vi "UHR-Fleezers Control (host) - 12.2.vi"() -> ()   [LabVIEW 2012] (continued)
  out "Y RF Amplitude Limits (%)":T16={"Minimum"=0.0, "Maximum"=50.0, "Increment"=1.0}
  in  "Manip. X?":bool=TRUE
  in  "Manip. Y?":bool
  in  "Force Manip Abort":bool
  out "Read cal error":errorcluster
  in  "DAQ Delay (ms)":u32=1000
  in  "Start Scan":bool
  in  "Scan axis":bool=TRUE
  in  "Osc. amp. (V)":dbl=5.0
  in  "Osc. center (V)":dbl=5.0
  in  "Osc. freq. (Hz) 2":dbl=1.0
  in  "MCL Mode":u16(ring) items=["Manual Positioning", "Sinusoidal Wave", "Linear Scan"]
  in  "Begin (V)":dbl
  in  "End (V)":dbl=10.0
  in  "N Points":dbl=20.0
  in  "Delay to Interlace (s)":dbl
  in  "Delayed Interlace Start":bool
  in  "Read Lateness and Rel Phase":bool
  out "Vec Mean of T1 T2":dbl[](array[numeric])=[nan, nan]
  in  "Cal read wait (s)":u32=5
  out "Time tether formed":timestamp=timestamp(3419012832.6319866 s since 1904-01-01)
  in  "Sample Chamber Stage Serial Port":refnum<visa-resource-name>="Sample-Stage-COM1"
  in  "Chemyx Syringe Pump Serial Port":refnum<visa-resource-name>="ASRL3::INSTR"
  in  "Limit Min (MHz)":dbl=10.0 caption="Min (MHz)"
  in  "Limit Max (MHz)":dbl=16.0 caption="Max (MHz)"
  in  "Limits Enable":bool=TRUE caption="Enable"
  out "AI labels":string[](array[string])=["T1 Y", "T1 X", "T1 Sum", "T2 Y", "T2 X", "T2 Sum", "T1 FB X", "T1 FB Sum", "T2 FB X", "T2 FB Sum", "PSD Y", "PSD X", "PSD Y Sum"]
  in  "Save Trap Pos. Data":bool=TRUE
  in  "Lower Ch. Cap.":bool
  in  "Top 3 Harvard Syringe Pump Serial Port":refnum<visa-resource-name>="Top-Pump3-COM4"
  # "After"
  # "During"
  # "Trap On?"
  # "BD Flow ON?"
  # "Samp Flow ON?"
  # "Trap Trig. Fl.?"
  # "Zero It"
  # "Floor it\n(e.g., hp unwinding)"
  # "1"
  # "2"
  # "Fl. Down"
  # "Fl. Up"
  # "Bead sep"
  # "Trap Display:"
  # "APD Display:"
  # "DAQ"
  # "Data Saving"
  # "Trap Manipulation"
  # "Bead Calibration"
  # "Bottom Pump (#1)"
  # "Central Sample Channels"
  # "Top Pump (#3)"
  # "Rate param is ul/h\nVolume param is ul"
  # "Chemyx Pump 2"
  # "Units: \n1 = ml/m\n2 = ml/h\n3 = ul/m\n4 = ul/h"
  # "X"
  # "Amp switch 1st is disabled in the fpga"
  # "Y"
  # "Oscillate Set 1 freq. (debugging)"
  # "BD 1"
  # "BD 2"
  # "AOD Raster Scan"
  # "Approx. trap separations"
  # "X"
  # "Y"
  # "FPGA\nreading"
  # "DMA\ntransfer"
  # "APD Gates"
  # "APD 2"
  # "APD 1"
  # "X"
  # "2D"
  # "Y"
  # "1D"
  # "Digital Out Control"
  # "Analog Out Control (Feedback Loop)"
  # "Laser Intensity Analog Input"
  # "Analog Out Control (Feedback Loop)"
  # "Digital Out Control"
  # "Laser Intensity Analog Input"
  # "Total AI Rates (NOT rates/trap)"
  # "(Samples/trap x Trap Sets)"
  # "(Samples/channel x\n8 if averaging (8 channels)\n4 if no averaging)"
  # "Trap 1"
  # "Trap 2"
  # "Flour./Trap 3"
  # "External Video Window"
  # "MCL Position Debugging"
  # "Temporary Control Storage\n(these used to be somewhere else, still want to keep them)"
  # "Y"
  # "X"
  # "Trap Position Difference Limits"
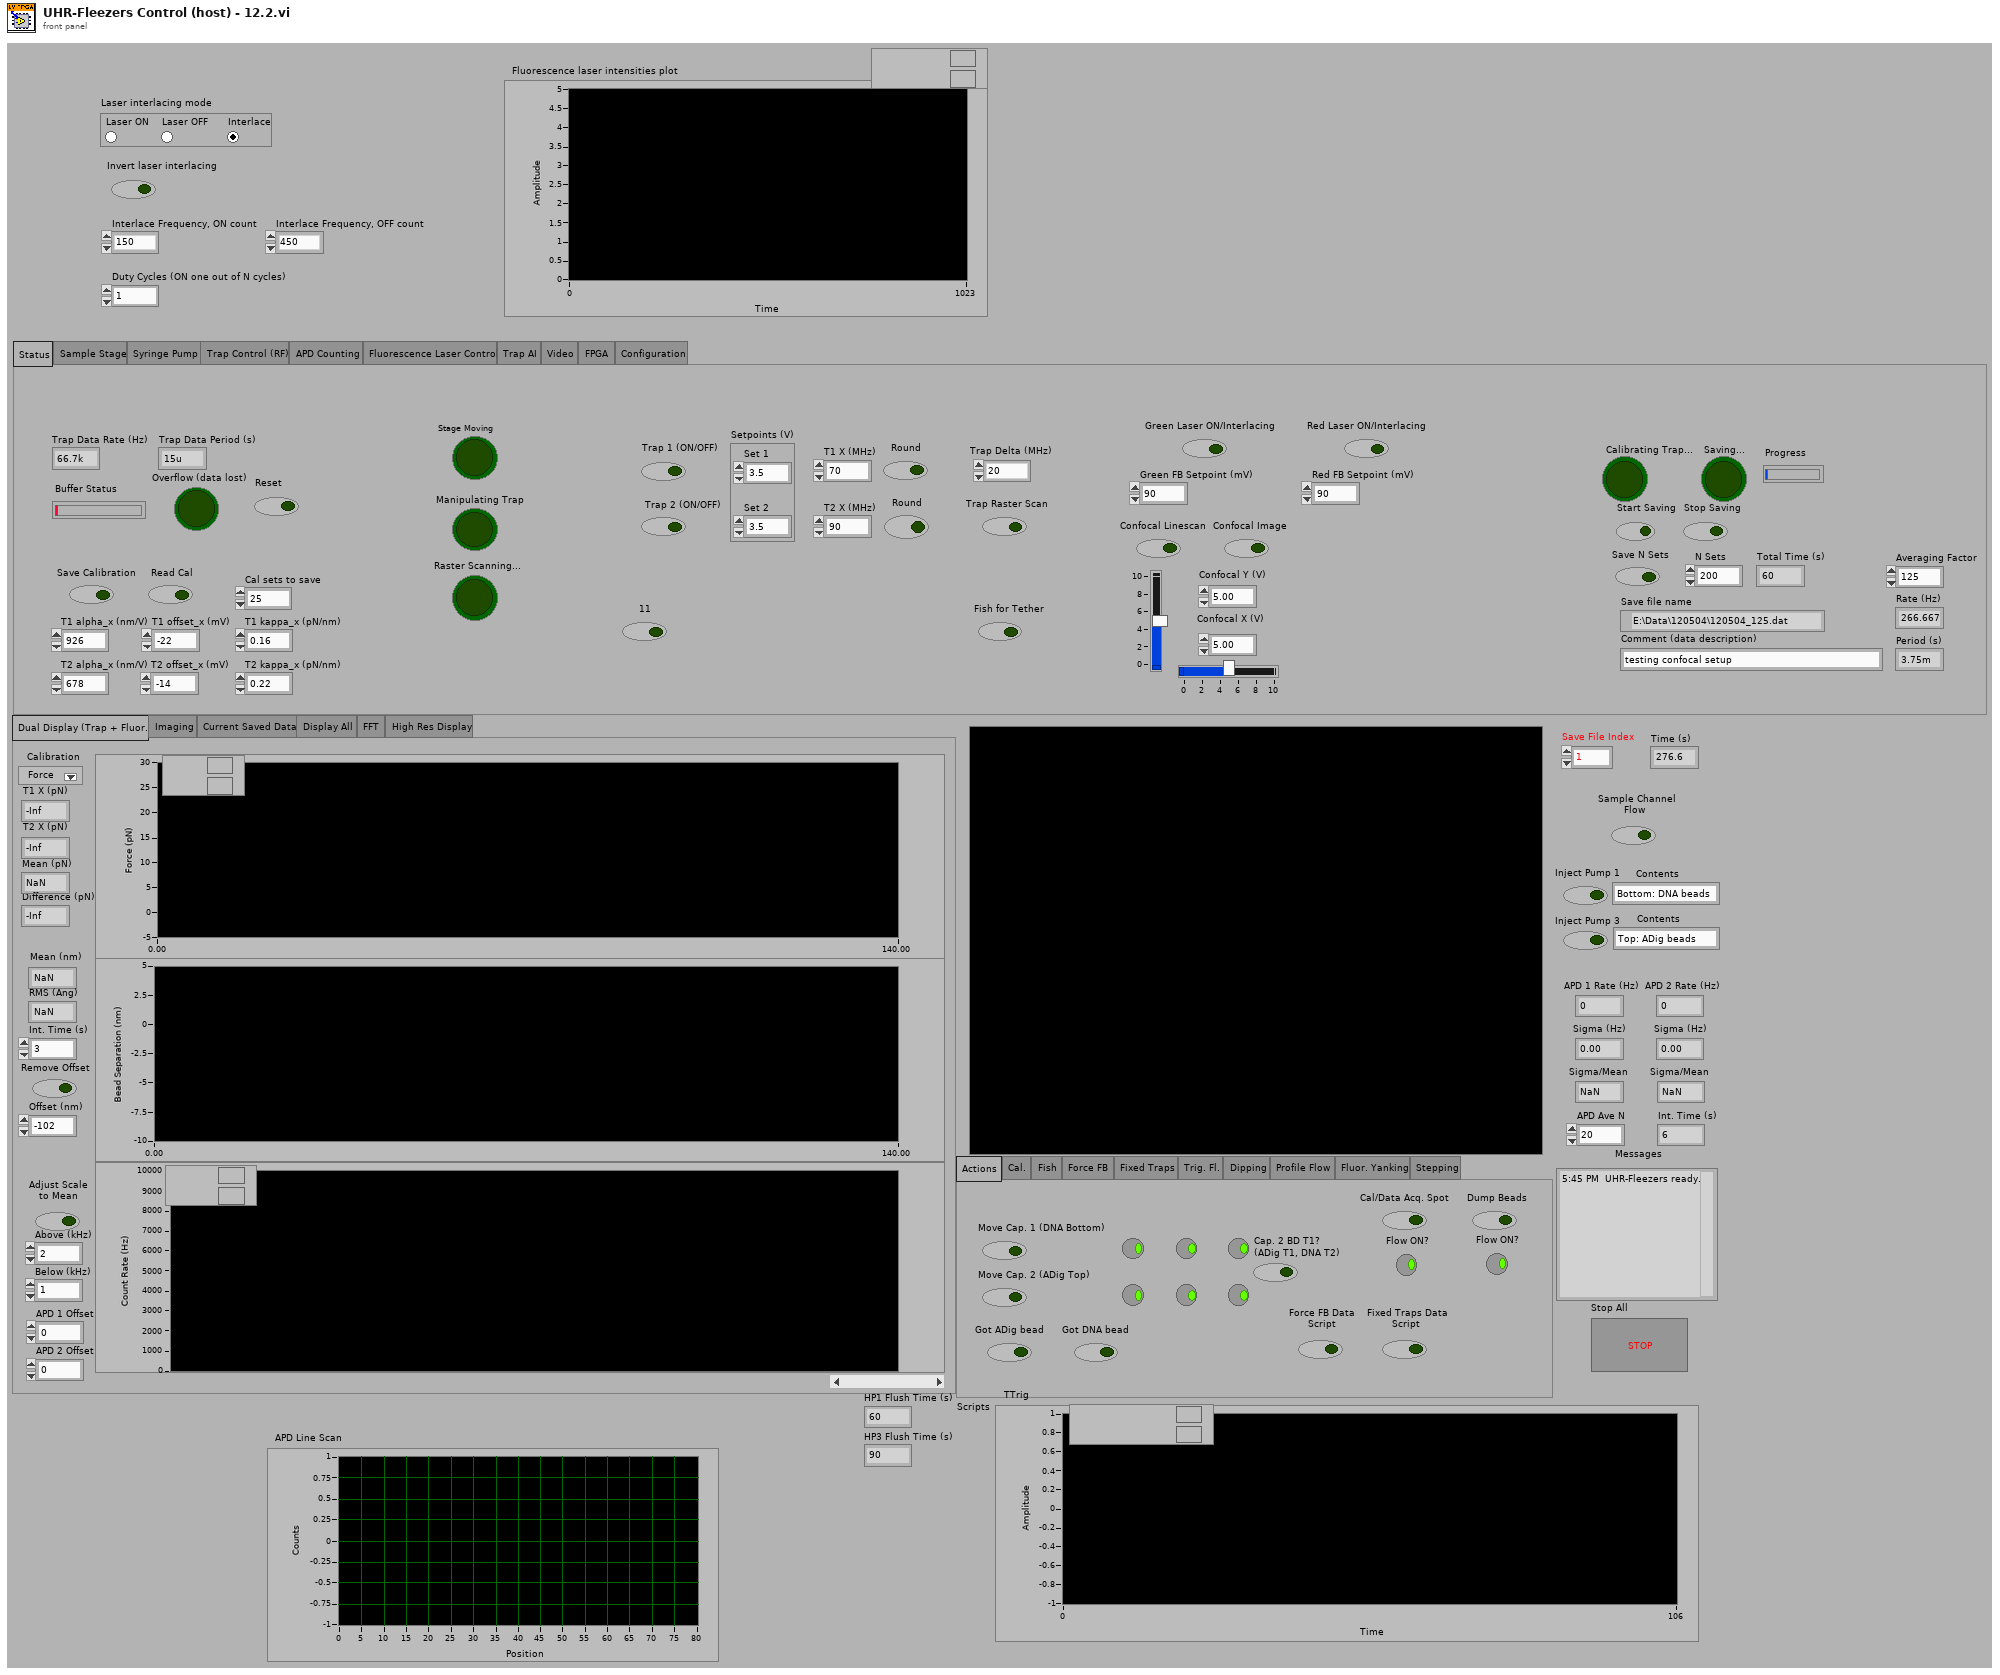
[diagram p1: front panel]
types:
  T1 = enum32{"Actions", "Cal.", "Fish", "Force FB", "Fixed Traps", "Trig. Fl.", "Dipping", "Profile Flow", "Fluor. Yanking", "Stepping"}
  T2 = typedef "IMAQ Image.ctl" = refnum<image>
  T3 = enum32{"Dual Display (Trap + Fluor.)", "Imaging", "Current Saved Data", "Display All", "FFT", "High Res Display"}
  T4 = enum32{"Status", "Sample Stage", "Syringe Pump", "Trap Control (RF)", "APD Counting", "Fluorescence Laser Control", "Trap AI", "Video", "FPGA", "Configuration"}
  T5 = cluster{"Pump 1":cluster{"Diameter (mm)":dbl, "Units":dbl, "Volume":dbl, "Rate":dbl}, "Pump 2":cluster{"Diameter (mm)":dbl, "Units":dbl, "Volume":dbl, "Rate":dbl}, "Pump 3":cluster{"Diameter (mm)":dbl, "Units":dbl, "Volume":dbl, "Rate":dbl}}
  T6 = enum32{"IR Laser Interlacing (Direct RF Board Control Method)", "AOD Raster Scan", "Feedback on Trap Intensity", "Feedback on Trap Position"}
  T7 = typedef "LVPoint32TypeDef.ctl" = cluster{"Horizontal":i32, "Vertical":i32}
  T8 = cluster{"Scan Range AOD (nm) 2":dbl, "Step Size AOD (nm) 2":dbl, "Scan Speed AOD (nm/s) 2":dbl, "Number of scans (AOD) 2":u16, "Label":string}[]
  T9 = cluster{"proportional gain (Kc)":i16, "integral gain (Kc*Ts/Ti)":i16, "derivative gain (Kc*Td/Ts)":i16}
  T10 = cluster{"Trap 1":fxp<+/-,16,1>, "Trap 2":fxp<+/-,16,1>}
  T11 = cluster{"proportional gain (Kc)":fxp<+/-,16,8>, "integral gain (Kc*Ts/Ti)":fxp<+/-,16,8>, "derivative gain (Kc*Td/Ts)":fxp<+/-,16,8>}
  T12 = cluster{"output high":fxp<+/-,16,1>, "output low":fxp<+/-,16,1>}
  T13 = cluster{"Set 1":fxp<+/-,16,1>, "Set 2":fxp<+/-,16,1>}
  T14 = enum32{"Shared Settings", "Green laser (532 nm)", "Red laser (633 nm)", "Blue laser (473 nm)"}
  T15 = cluster{"Set 1":bool, "Set 2":bool, "Set 3":bool}
  T16 = typedef "LVMinMaxIncTypeDef.ctl" = cluster{"Minimum":dbl, "Maximum":dbl, "Increment":dbl}
  T17 = typedef "Image Type" = u32
  T18 = typedef "nirio_resource_hc.ctl" = tag
  T19 = typedef "openfpgaref.8.6.ctl" = refnum<k20>
  T20 = cluster{"New Image":T2, "New Image":T2, "New Image":T2, "New Image":T2}
  T21 = typedef "XDNodeRunTimeDep.lvlib/timing_clust.ctl" = cluster{"Expected End [f-1]":u64, "Actual End [f-1]":u64, "Finished Late? [f-1]":bool, "Expected End [i-1]":u64, "Actual End [i-1]":u64, "Finished Late? [i-1]":bool, "Expected Start [i]":u64, "Actual Start [i]":u64, "Expected Start [f]":u64, "Actual Start [f]":u64, "Source Name":string, "Structure Name":string, "Period":i64, "Deadline":i64, "Offset":i64, "Start":i64, "Priority":i32, "Timeout":i32, "Mode":T22, "Wakeup Reason":T23, "Error":errorcluster, "Source Type":string, "Secondary Source Type":string, "Global End Time":u64, "Global Start Time":u64, "Frame Duration":u64, "Iteration Duration":u64, "Assigned CPU":i32, "I/O Scan Engine Mode":u32}
  T22 = typedef "XDNodeRunTimeDep.lvlib/nitl_modes.ctl" = enum32{"No Change", "Process missed periods, maintain original phase", "Discard missed periods, maintain original phase", "Process missed periods, ignore original phase", "Discard missed periods, ignore original phase"}
  T23 = typedef "XDNodeRunTimeDep.lvlib/wakeup.ctl" = enum32{"Normal", "Aborted", "Asynchronous wakeup", "Timing source error", "Timed loop error", "Timeout"}
  T24 = cluster{"Left":i32, "Top":i32, "Width":u32, "Height":u32}
  T25 = cluster{cluster{"Left":i32, "Top":i32, "Width":u32, "Height":u32}}[]
  T26 = enum32{"setting", "request", "request control", "info", "statistics", "system settings", "I/O sub system", "HRT control", "camera descriptions", "device specific data", "event sub system settings", "event sub system results", "image memory manager"}
  T27 = typedef "AviRefnum.ctl" = refnum<k1>
  T28 = typedef "imagedata.ctl" = cluster{"image type":i32, "image depth":i32, "image":u8[], "mask":u8[], "colors":u32[], "Rectangle":cluster{"left":i16, "top":i16, "right":i16, "bottom":i16}}
  T29 = enum32{"Normal Display", "Dual Display (APD)", "FFT", "High Res Display"}
  T30 = cluster{"Origin Pixel":cluster{"X":sgl, "Y":sgl}, "Angle Relative to Horizontal (deg)":sgl, "Axis Reference":u32}
  T31 = typedef "Simple Grid Descriptor" = cluster{"X Step":sgl, "Y Step":sgl, "Unit":T32}
  T32 = typedef "Image Unit" = enum32{"Undefined", "Angström", "Micrometer", "Millimeter", "Centimeter", "Meter", "Kilometer", "Microinch", "Inch", "Feet", "Nautical miles", "Standard miles", "Steps"}
  T33 = cluster{"averaging mode":u16, "weighting mode":u16, "number of averages":u32}
  T34 = cluster{"dB On (F)":bool, "unwrap phase (F)":bool, "convert to degree (F)":bool}
  T35 = enum16{"open", "replace", "create", "open or create", "replace or create", "replace or create with confirmation"}
  T36 = enum16{"big-endian, network order", "native, host order", "little-endian"}
  T37 = cluster{string, string, string, string, string, string, string, string}
  T38 = cluster{string, string, string, string, string, string, string, string, string, string, string, string}
  T39 = cluster{string, string, string, string, string, string, string, string, string, string, string, string, string}
  T40 = cluster{string, string, string, string, string, string, string, string, string, string, string, string, string, string}
  T41 = cluster{"BD 1 Frequency 1 (MHz)":dbl, "BD 1 Frequency 2 (MHz)":dbl}
  T42 = cluster{"f0":dbl, "df":dbl, "magnitude":dbl[]}[][]
  T43 = cluster{"Scan Range AOD (nm) 2":dbl, "Step Size AOD (nm) 2":dbl, "Scan Speed AOD (nm/s) 2":dbl, "Number of scans (AOD) 2":u16, "Label":string}
  T44 = cluster{"[0]":dbl, "[1]":dbl, "[2]":dbl, "[3]":dbl, "[4]":dbl, "[5]":dbl}
  T45 = cluster{"Diameter (mm)":dbl, "Units":dbl, "Volume":dbl, "Rate":dbl}
diagram:
  w58 = u16 20 items=["1.0"=10, "1.5"=15, "2.0"=20] ("stop bits (10: 1 bit)")
  w61 = u16 20 items=["1.0"=10, "1.5"=15, "2.0"=20] ("stop bits (10: 1 bit)")
  w112 = u16 20 items=["1.0"=10, "1.5"=15, "2.0"=20] ("stop bits (10: 1 bit)")
  w119 = T17 2 items=["Grayscale (U8)", "Grayscale (I16)", "Grayscale (SGL)", "Complex (CSG)", "RGB (U32)", "HSL (U32)", "RGB (U64)", "Grayscale (U16)"] ("Image Type")
  w246 = 10.0 ("y")
  w245 = 32767.0 ("y")
  w261 = 6.0  # clock mult.
  w262 = 49152000.0  # TCXO frequ.
  # "I don't think you need to do this.\nEverytime you want to adjust phase you always set this anyway.\nSince we removed the separate +/- controls.\n\nHaven't added for added fl lasers.  Should remove this code."
  # "Bottom 1 Harvard"
  # "Top 3 Harvard"
  # "Center Harvard"
  # "Bottom 1 Harvard"
  # "Top 3 Harvard"
  # "Center Harvard"
  n1 = Build Array("DIO count 1 (ticks)", "DIO count 2 (ticks)", "DIO count 3 (ticks)") -> (w166:u32[])
  n2 = local read "AO1"() -> (w240:dbl)
  n3 = local read "AO2"() -> (w239:dbl)
  n4 = local read "Scan Increment (MHz)"() -> (w257:dbl)
  n5 = local read "Continuous MCL Scanning"() -> (w227:bool)
  n6 = local read "Fast Scan Dir"() -> (w226:bool)
  n7 = local read "Number of scans (MCL)"() -> (w228:u64)
  n8 = property on="AI Count (ticks)" class="DigNum (strict)"("Val(Sgnl)"="AI Count (ticks)") -> ()  [unwired: 2 in, 2 out]
  n9 = Multiply(x=w240, y=w245) -> (x*y=w242:dbl)
  n10 = Multiply(x=w239, y=w245) -> (x*y=w244:dbl)
  n11 = Divide(x=w242, y=w246) -> (x/y=w241:dbl)
  n12 = Divide(x=w244, y=w246) -> (x/y=w243:dbl)
  n13 = To Word Integer(number=w241) -> (16bit integer=w238:i16)
  n14 = To Word Integer(number=w243) -> (16bit integer=w237:i16)
  n15 = Not(x=w226) -> (.not. x?=w221:bool)
  n16 = local read "Cycles/step (MCL)"() -> (w229:u64)
  n17 = Multiply(x=w257, y=1000.0) -> (x*y=w264:dbl)
  n18 = local read "Scan steps (MCL)"() -> (w230:u64)
  n19 = local write "Trap Pos FIFO Timeout"(u16 0 ("Trap Pos FIFO Timeout")) -> ()
  n20 = local read "Desired Scan Incr (V)"() -> (w232:dbl)
  n21 = Scale By Power Of 2(n=48, x=w264) -> (x*2^n=w265:dbl)
  n22 = Unbundle By Name(cluster{"output high":i16, "output low":i16} {"output high"=3000, "output low"=0} ("FB output range 1")) -> ("output high"=w38:i16, "output low"=w37:i16)
  n23 = Multiply(x=w262, y=w261) -> (x*y=w260:dbl)
  n24 = Divide(x=w265, y=w260) -> (x/y=w259:dbl)
  n25 = local read "Setpoints (V)"() -> (w276:cluster{"Set 1":dbl, "Set 2":dbl})
  n26 = To Quad Integer(1:w259) -> (0:w256:i64)
  n27 = Divide(x=40000000.0, y="AI Count (ticks)") -> (x/y=w217:dbl)
  n28 = Multiply(x=w232, y=32767.0) -> (x*y=w234:dbl)
  n29 = local read "Trap Intensity PID Gains"() -> (w271:T9)
  n30 = local read "Number Interlace Sets"() -> (w159:u8)
  n31 = Split 1D Array(array=w166, index=w159) -> (first subarray=w168:u32[])  [unwired: 1 out]
  n32 = Add Array Elements(numeric array=w168) -> (sum=w167:u32)
  n33 = local read "# Samples/channel"() -> (w249:u32)
  n34 = local read "Number of F/B Scans (AOD)"() -> (w250:u16)
  n35 = local read "Not-Interlacing Set"() -> (w158:enum32{"Set 1", "Set 2", "Set 3"})
  n36 = To Unsigned Byte Integer(number=w158) -> (unsigned 8bit integer=w164:u8)
  n37 = Index Array(array=w166, index=w164) -> (element=w165:u32)
  n38 = local read "Feedback On/Off"() -> (w279:cluster{"Set 1":bool, "Set 2":bool})
  n39 = local read "Scan steps (AOD)"() -> (w255:u64)
  n40 = local read "All FB On/Off"() -> (w280:bool)
  n41 = local read "Cycles/step (AOD)"() -> (w254:u64)
  n42 = local write "AI rate (Hz)"(w217) -> ()
  n43 = Divide(x=w234, y=10.0) -> (x/y=w233:dbl)
  n44 = Multiply(x=w255, y=w254) -> (x*y=w253:u64)
  n45 = Unbundle By Name(w271) -> ("proportional gain (Kc)"=w42:i16, "integral gain (Kc*Ts/Ti)"=w41:i16, "derivative gain (Kc*Td/Ts)"=w40:i16)
  n46 = Multiply(x=3276.7, y=w276) -> (x*y=w275:cluster{"Set 1":dbl, "Set 2":dbl})
  n47 = xnode "Open FPGA VI Reference"("resource name"=T18 "750kHzDAQ") -> ("FPGA VI Reference Out"=w270:T19, "error out"=w269:errorcluster)  [unwired: 1 in]
  n48 = To Word Integer(number=w233) -> (16bit integer=w231:i16)
  n49 = Multiply(x=w253, y=u64 2) -> (x*y=w251:u64)
  n50 = Divide(x=w217, y="FPGA Ave.") -> (x/y=w218:dbl)
  n51 = To Word Integer(number=w275) -> (16bit integer=w274:cluster{"Set 1":i16, "Set 2":i16})
  n52 = Multiply(x=w251, y=w250) -> (x*y=w248:u64)
  n53 = local read "Sets to FIFO (Traps)"() -> (w46:T15)
  n54 = local write "Ave. Rate (Hz)"(w218) -> ()
  n55 = Divide(x=w248, y=w249) -> (x/y=w247:dbl)
  n56 = Unbundle By Name(w274) -> ("Set 1"=w273:i16, "Set 2"=w272:i16)
  n57 = local read "2D or 1D Scan"() -> (w178:bool)
  n58 = local write "Data points/scans"(w248) -> ()
  n59 = local read "Scan BD"() -> (w266:bool)
  n60 = And(x=w279, y=w280) -> (x .and. y?=w278:cluster{"Set 1":bool, "Set 2":bool})
  n61 = local write "Data points/scan (f/b)"(w251) -> ()
  n62 = Reciprocal(x=w218) -> (1/x=w219:dbl)
  n63 = local read "N Acq Sets (Traps + Fl.)"() -> (w210:i16)
  n64 = local write "N sets should be saved"(w247) -> ()
  n65 = xnode "Invoke Method"("FPGA VI Reference In"=w270, "error in"=w269) -> ("FPGA VI Reference Out"=w177:T19, "error out"=w186:errorcluster)
  n66 = Unbundle By Name(w278) -> ("Set 1"=w282:bool, "Set 2"=w281:bool)
  n67 = local read "Interlace"() -> (w160:bool)
  n68 = Select(t=w167, s=w160, f=w165) -> (s? t:f=w157:u32)
  n69 = local write "Update Count (MCL)"(w157) -> ()
  n70 = local write "Total Counts (ticks)"(w157) -> ()
  n71 = local write "Ave. Period (s)"(w219) -> ()
  n72 = Unbundle By Name(w46) -> ("Set 1"=w45:bool, "Set 2"=w44:bool, "Set 3"=w43:bool)
  n73 = property on="2D or 1D Scan" class="Bool (strict)"("Val(Sgnl)"=w178) -> ()  [unwired: 2 in, 2 out]
  n74 = local read "Interlace Frequency, OFF count"() -> (w4:u32)
  n75 = local read "Interlace Frequency, ON count"() -> (w5:u32)
  n76 = local read "APD Gate OFF Count"() -> (w84:u32)
  n77 = local read "APD Gate ON Count"() -> (w80:u32)
  n78 = xnode "Read/Write Control"("FPGA VI Reference In"=w176, "error in"=w186, "ai count"="AI Count (ticks)", "Interlace ON/OFF"=w160, "Number Interlace Cycles"=w159, "Set 1"=w45, "Set 2"=w44, "Set 3"=w43, "FB On/Off Set 1"=w282, "FB On/Off Set 2"=w281, "Interlace Off Parameters"=w158, "FB Setpoint Set 1"=w273, "FB Setpoint Set 2"=w272, "P1"=w42, "I1"=w41, "D1"=w40, "FB1 output high"=w38, "FB1 output low"=w37, "Cycles per step"=w254, "Scan BD"=w266, "Number of scans"=w250, "Scan steps"=w255, "Scan freq.  increment"=w256, "AO1"=w238, "AO2"=w237, "Scan freq.  increment (MCL)"=w231, "Scan steps (MCL)"=w230, "Cycles per step (MCL)"=w229, "Number of scans (MCL)"=w228, "MCL count"=w157, "Cont. Scan (MCL)"=w227, "MCL Scan Axis"=w221, "1D or 2D Scan?"=w178, "N of AI1 Int Acq Sets"=w210, "Amp switch delay"="Amp switch delay", "Swap F1 and F2"="Swap F1 and F2", "APD to FIFO"=FALSE, "DIO count 1 (ticks)"="DIO count 1 (ticks)", "DIO count 2 (ticks)"="DIO count 2 (ticks)", "DIO count 3 (ticks)"="DIO count 3 (ticks)") -> ("FPGA VI Reference Out"=w90:T19, "error out"=w88:errorcluster)  [unwired: 1 in]
  n79 = local read "Duty Cycles (ON one out of N cycles)"() -> (w86:u32)
  n80 = local read "APD Integration Time (s)"() -> (w72:dbl)
  n81 = local read "DMA Update Period (s)"() -> (w71:dbl)
  n82 = Add(x=w80, y=w84) -> (x+y=w82:u32)
  n83 = Add(x=w5, y=w4) -> (x+y=w85:u32)
  n84 = local read "Green Laser ON/Interlacing"() -> (w155:bool)
  n85 = local read "Laser interlacing mode"() -> (w156:enum32{"Laser ON", "Laser OFF", "Interlace"})
  n86 = local read "Trap Pos. FB Range"() -> (w36:T12)
  n87 = local read "Trap Pos. FB Gains"() -> (w35:T11)
  n88 = Multiply(x=w82, y=w86) -> (x*y=w83:u32)
  n89 = Multiply(x=w86, y=w85) -> (x*y=w3:u32)
  n90 = Reciprocal(x=w72) -> (1/x=w69:dbl)
  n91 = Multiply(x=w72, y=40000000.0) -> (x*y=w68:dbl)
  n92 = Divide(x=w71, y=w72) -> (x/y=w74:dbl)
  n93 = Multiply(x="Current When FB OFF (%)", y=655.35) -> (x*y=w146:dbl)
  n94 = local read "Invert laser interlacing"() -> (w13:bool)
  n95 = local read "Trap Pos. AI1 X Pre-scale"() -> (w100:u16)
  n96 = local read "Invert APD Gate"() -> (w78:bool)
  n97 = Multiply(x="Green FB Setpoint (mV)", y=3.2767) -> (x*y=w143:dbl)
  n98 = local read "APD Gate"() -> (w77:enum32{"ON", "OFF", "Interlace"})
  n99 = local read "Trap Pos FB Int Count"() -> (w94:u16)
  n100 = Subtract(x=w83, y=w80) -> (x-y=w81:u32)
  n101 = local write "Green FB Count"(w3) -> ()
  n102 = local write "APD Acq Rate (Hz)"(w69) -> ()
  n103 = local read "Differential FB?"() -> (w63:bool)
  n104 = To Unsigned Long Integer(number=w68) -> (unsigned 32bit integer=w66:u32)
  n105 = local read "Neg. TTrig FPGA"() -> (w65:bool)
  n106 = local write "Green FB Count"(w3) -> ()
  n107 = Multiply(x=2.0, y=w74) -> (x*y=w73:dbl)
  n108 = Multiply(x="Red FB Setpoint (mV)", y=3.2767) -> (x*y=w22:dbl)
  n109 = To Unsigned Word Integer(number=w146) -> (unsigned 16bit integer=w144:u16)
  n110 = Subtract(x=w3, y=w5) -> (x-y=w79:u32)
  n111 = Multiply(x="Current When RI FB OFF (%)", y=655.35) -> (x*y=w18:dbl)
  n112 = local write "APD Samples/FIFO Acq."(w74) -> ()
  n113 = To Word Integer(number=w143) -> (16bit integer=w141:i16)
  n114 = Unbundle By Name("Green FB Gains") -> ("proportional gain (Kc)"=w27:i16, "integral gain (Kc*Ts/Ti)"=w26:i16, "derivative gain (Kc*Td/Ts)"=w25:i16)
  n115 = local write "APD Elements/DMA read"(w73) -> ()
  n116 = case shown="False" w155 {
    tunnel: w156 -> [_ w308]
    tunnel: [enum32{"Laser ON", "Laser OFF", "Interlace"}."Laser OFF" ("Green laser mode") w308] -> w12
    frame False {
    }
    frame True {
    }
  }
  n117 = local write "APD Int. Count"(w66) -> ()
  n118 = To Word Integer(number=w22) -> (16bit integer=w19:i16)
  n119 = Unbundle By Name("Red FB Gains") -> ("proportional gain (Kc)"=w10:i16, "integral gain (Kc*Ts/Ti)"=w9:i16, "derivative gain (Kc*Td/Ts)"=w8:i16)
  n120 = Unbundle By Name(w35) -> ("proportional gain (Kc)"=w31:fxp<+/-,16,8>, "integral gain (Kc*Ts/Ti)"=w30:fxp<+/-,16,8>, "derivative gain (Kc*Td/Ts)"=w29:fxp<+/-,16,8>)
  n121 = To Unsigned Word Integer(number=w18) -> (unsigned 16bit integer=w15:u16)
  n122 = Unbundle By Name(w36) -> ("output high"=w34:fxp<+/-,16,1>, "output low"=w32:fxp<+/-,16,1>)
  n123 = local read "Trap Pos FB Monitor\nT1 or T2"() -> (w105:bool)
  n124 = local read "APD 1 AO Mult."() -> (w76:i16)
  n125 = local read "Trap Pos FB Negate Action"() -> (w104:bool)
  n126 = local read "APD 2 AO Mult."() -> (w75:i16)
  n127 = local read "Trap Pos. FB Offset Factor"() -> (w103:i64)
  n128 = local read "Trap Pos. FB Mult Factor"() -> (w102:i64)
  n129 = xnode "Read/Write Control"("FPGA VI Reference In"=w90, "error in"=w88, "Invert APD Gate"=w78, "APD Gate ON Count"=w80, "APD Gate OFF Count"=w81, "APD Acq Rate Count"=w66, "APD Gate Operating Mode"=w77, "APD 1 AO scale factor"=w76, "APD 2 AO scale factor"=w75, "Green interlace ON count"=w5, "Green interlace OFF count"=w79, "Green interlace ON count 2"=w5, "Green interlace OFF count 2"=w79, "Green FB Count"=w3, "Red interlace OFF count"=w4, "Red interlace ON count"=w5, "Red FB Count"=w3, "Red interlace OFF count 2"=w4, "Red interlace ON count 2"=w5) -> ("FPGA VI Reference Out"=w89:T19, "error out"=w87:errorcluster)
  n130 = xnode "Read/Write Control"("FPGA VI Reference In"=w89, "error in"=w87, "Invert GI 2"=w13, "Operating Mode 2"=w12, "P3"=w27, "I3"=w26, "D3"=w25, "Green FB Setpoint"=w141, "Green FB On/Off"="Green FB On/Off", "Current Out"=w144, "Green int current ON count adj"="Green int current ON count adj", "Operating Mode"=w12, "Invert GI"=w13, "Trap Pos FB Monitor T1 or T2"=w105, "Trap Pos FB Negate Action"=w104, "Trap Pos. FB Offset Factor"=w103, "Trap Pos. FB Mult Factor"=w102, "Force feedback"=FALSE, "AI1 X Scale"=w100, "Trap Pos to FIFO"=TRUE, "Trap Pos FB Int Count"=w94, "TTrig Negate Pos"=w65, "FB Trig Integrate"="FB Trig Integrate", "Diff FB Measurement?"=w63, "Negate Diff?"="Negate Diff?", "P2"=w31, "I2"=w30, "D2"=w29, "FB2 output high"=w34, "FB2 output low"=w32, "Red FB Setpoint"=w19, "RI Current Out"=w15, "Red int current ON count adj"="Red int current ON count adj", "Red Laser Operating Mode"=w12, "RI Operating Mode 2"=w12, "Invert RI 2"=w13, "Invert RI"=w13, "P4"=w10, "I4"=w9, "D4"=w8, "Red FB On/Off"="Red FB On/Off") -> ("FPGA VI Reference Out"=w153:T19, "error out"=w154:errorcluster)
  n131 = xnode "Invoke Method"("FPGA VI Reference In"=w153, "error in"=w154, "Requested Depth"="Trap AI FIFO Depth") -> ("FPGA VI Reference Out"=w108:T19, "error out"=w107:errorcluster)  [unwired: 1 out]
  n132 = xnode "Invoke Method"("FPGA VI Reference In"=w108, "error in"=w107, "Requested Depth"="Trap Position FIFO Depth") -> ("FPGA VI Reference Out"=w96:T19, "error out"=w95:errorcluster)  [unwired: 1 out]
  n133 = flat-sequence {
    tunnel: w177 -> [w313]
    tunnel: [w313] -> w176
    tunnel: [w312] -> w175
    tunnel: [w311] -> w174
    tunnel: [w309] -> w172
    tunnel: [w310] -> w173
    frame #0 {
      w310 = T16 {"Minimum"=0.0, "Maximum"=40.0, "Increment"=1.0} ("Min Max Inc")
      w309 = T16 {"Minimum"=0.0, "Maximum"=50.0, "Increment"=1.0} ("Data Entry Limits")
      w312 = T16 {"Minimum"=60.0, "Maximum"=90.0, "Increment"=1.0} ("Min Max Inc")
      w311 = T16 {"Minimum"=0.0, "Maximum"=50.0, "Increment"=1.0} ("Data Entry Limits")
      n134 = property on="BD 2 Frequency 1 (MHz)" class="DigNum (strict)"("Data Range"=w310) -> ()  [unwired: 2 in, 2 out]
      n135 = property on="BD 2 Frequency 3 (MHz)" class="DigNum (strict)"("Data Range"=w310) -> ()  [unwired: 2 in, 2 out]
      n136 = property on="BD 2 Frequency 2 (MHz)" class="DigNum (strict)"("Data Range"=w310) -> ()  [unwired: 2 in, 2 out]
      n137 = property on="BD 1 Frequency 1 (MHz)" class="DigNum (strict)"("Data Range"=w312) -> ()  [unwired: 2 in, 2 out]
      n138 = property on="BD 1 Frequency 2 (MHz)" class="DigNum (strict)"("Data Range"=w312) -> ()  [unwired: 2 in, 2 out]
      n139 = property on="BD 1 Frequency 3 (MHz)" class="DigNum (strict)"("Data Range"=w312) -> ()  [unwired: 2 in, 2 out]
      n140 = property on="BD 2 Amplitude 1 (%)" class="DigNum (strict)"("Data Range"=w309) -> ()  [unwired: 2 in, 2 out]
      n141 = property on="BD 2 Amplitude 2 (%)" class="DigNum (strict)"("Data Range"=w309) -> ()  [unwired: 2 in, 2 out]
      n142 = property on="BD 2 Amplitude 3 (%)" class="DigNum (strict)"("Data Range"=w309) -> ()  [unwired: 2 in, 2 out]
      n143 = property on="BD 1 Amplitude 3 (%)" class="DigNum (strict)"("Data Range"=w311) -> ()  [unwired: 2 in, 2 out]
      n144 = property on="BD 1 Amplitude 2 (%)" class="DigNum (strict)"("Data Range"=w311) -> ()  [unwired: 2 in, 2 out]
      n145 = property on="BD 1 Amplitude 1 (%)" class="DigNum (strict)"("Data Range"=w311) -> ()  [unwired: 2 in, 2 out]
      "X RF Frequency Limits (MHz)" <- w312
      "X RF Amplitude Limits (%)" <- w311
      "Y RF Amplitude Limits (%)" <- w309
      "Y RF Frequency Limits (MHz)" <- w310
    }
  }
  n146 = xnode "Invoke Method"("FPGA VI Reference In"=w96, "error in"=w95) -> ("FPGA VI Reference Out"=w185:T19, "error out"=w184:errorcluster)  [unwired: 1 in]
  n147 = flat-sequence "Initial FPGA Loop Relative Phase Adjustment" {
    tunnel: "Initial Phase Adjustment (AI1)" -> [w327]
    tunnel: "Initial Phase Adjustment (GI)" -> [w326]
    tunnel: w185 -> [w325]
    tunnel: w184 -> [w324]
    tunnel: "Initial Phase Adj. (MCL)" -> [w323]
    tunnel: [w328] -> w194
    tunnel: [w322] -> w190
    tunnel: "Initial Phase Adjustment (APD Acq)" -> [w321]
    tunnel: "Initial Phase Adjustment (APD 1 Gate)" -> [w320]
    tunnel: "Initial Phase Adjustment (Green FB)" -> [w319]
    tunnel: "Initial Phase Adjustment (GI) 2" -> [w318]
    tunnel: "Initial Phase Adjustment (APD 2 Gate)" -> [w317]
    tunnel: "Initial Phase Adjustment (RI)" -> [w316]
    tunnel: "Initial Phase Adjustment (RI) 2" -> [w315]
    tunnel: "Initial Phase Adjustment (RI FB)" -> [w314]
    tunnel: w194 -> [w330]
    tunnel: [w331] -> w191
    tunnel: w190 -> [w331]
    tunnel: [w330] -> w189
    tunnel: w191 -> [w334]
    tunnel: w189 -> [w333]
    tunnel: [w336] -> w188
    tunnel: [w335] -> w187
    tunnel: [w338] -> w192
    tunnel: [w339] -> w193
    tunnel: w188 -> [w339]
    tunnel: w187 -> [w338]
    frame #0 {
      n148 = xnode "Read/Write Control"("FPGA VI Reference In"=w325, "error in"=w324, "Phase count adjustment"=w327, "Phase count adjustment (GI)"=w326, "Phase count adjustment (MCL)"=w323, "Phase Count Adjustment (APD Acq)"=w321, "Phase count adjustment (APD 1 Gate)"=w320, "Phase count adjustment (APD 2 Gate)"=w317, "Phase count adjustment (Green FB)"=w319, "Phase count adjustment (GI) 2"=w318, "Phase count adjustment (RI)"=w316, "Phase count adjustment (RI) 2"=w315, "Phase count adjustment (Red FB)"=w314) -> ("FPGA VI Reference Out"=w322:T19, "error out"=w328:errorcluster)
    }
    frame #1 {
      n149 = Wait (ms)(milliseconds to wait=u32 100) -> ()  [unwired: 1 out]
    }
    frame #2 {
      w332 = TRUE
      n150 = xnode "Read/Write Control"("FPGA VI Reference In"=w334, "error in"=w333, "+ phase"=w332, "+ phase (GI)"=w332, "+ phase (MCL)"=w332, "+ phase (APD Acq)"=w332, "+ phase (APD 1 Gate)"=w332, "+ phase (APD 2 Gate)"=w332, "+ phase (Green FB)"=w332, "+ phase (GI) 2"=w332, "+ phase (RI)"=w332, "+ phase (RI) 2"=w332) -> ("FPGA VI Reference Out"=w335:T19, "error out"=w336:errorcluster)
    }
    frame #3 {
      n151 = Wait (ms)(milliseconds to wait=u32 100) -> ()  [unwired: 1 out]
    }
  }
  n152 = local read "Phase adj. (Green FB)"() -> (w169:i16)
  n153 = local read "Phase adj. (GI) 2"() -> (w147:i16)
  n154 = local read "Phase adjust (MCL)"() -> (w222:i16)
  n155 = local read "Phase adj. (AI1)"() -> (w224:i16)
  n156 = local read "Phase adj. (GI)"() -> (w223:i16)
  n157 = xnode "Read/Write Control"("FPGA VI Reference In"=w192, "error in"=w193, "Phase count adjustment"=w224, "Phase count adjustment (GI)"=w223, "Phase count adjustment (MCL)"=w222, "Phase Count Adjustment (APD Acq)"="Phase Adj. (APD Acq)", "Phase count adjustment (APD 1 Gate)"="Phase Adj. (APD 1 Gate)", "Phase count adjustment (APD 2 Gate)"="Phase Adj. (APD 2 Gate)", "Phase count adjustment (Green FB)"=w169, "Phase count adjustment (GI) 2"=w147) -> ("FPGA VI Reference Out"=w133:T19, "error out"=w199:errorcluster)
  n158 = call "Initialize RF boards - interlace 3.vi"("error in"=w199, "FPGA VI Reference In"=w133) -> ("error out"=w197:errorcluster, "FPGA VI Reference Out"=w198:T19)
  n159 = call "set RF board frequency - interlace.vi"("Board 2 Frequency Limits"=w173, "Board 1 Frequency Limits"=w175, "error in"=w197, "FPGA VI Reference In"=w198, "Board 2 Frequency 3 (MHz)"="BD 2 Frequency 3 (MHz)", "Board 1 Frequency 3 (MHz)"="BD 1 Frequency 3 (MHz)", "Board 2 Frequency 2 (MHz)"="BD 2 Frequency 2 (MHz)", "Board 2 Frequency 1 (MHz)"="BD 2 Frequency 1 (MHz)", "Board 1 Frequency 2 (MHz)"="BD 1 Frequency 2 (MHz)", "Board 1 Frequency 1  (MHz)"="BD 1 Frequency 1 (MHz)") -> ("error out"=w297:errorcluster, "FPGA VI Reference Out"=w298:T19)
  n160 = call "set RF board amplitude - interlace.vi"("Board 2 Amplitude Limits"=w172, "Board 1 Amplitude Limits"=w174, "error in"=w297, "FPGA VI Reference In"=w298, "Board 2 Amplitude 3 (%)"="BD 2 Amplitude 3 (%)", "Board 1 Amplitude 3 (%)"="BD 1 Amplitude 3 (%)", "Board 2 Amplitude 2 (%)"="BD 2 Amplitude 2 (%)", "Board 2 Amplitude 1 (%)"="BD 2 Amplitude 1 (%)", "Board 1 Amplitude 2 (%)"="BD 1 Amplitude 2 (%)", "Board 1 Amplitude 1 (%)"="BD 1 Amplitude 1 (%)") -> ("error out"=w285:errorcluster, "FPGA VI Reference Out"=w286:T19)
  n161 = flat-sequence {
    tunnel: w286 -> [w349]
    tunnel: w285 -> [w348]
    tunnel: [w347] -> w290
    tunnel: [w346] -> w289
    tunnel: [w353] -> w288
    tunnel: w290 -> [w353]
    tunnel: [w352] -> w287
    tunnel: w289 -> [w352]
    tunnel: w288 -> [w362]
    tunnel: w287 -> [w361]
    tunnel: [w360] -> w52
    tunnel: [w359] -> w97
    frame #0 {
      w340 = FALSE ("Retract Pump 3")
      n162 = local read "Trap 1 (ON/OFF)"() -> (w341:bool)
      n163 = xnode "Read/Write Control"("FPGA VI Reference In"=w349, "error in"=w348, "Direct RF Box  Communication"=FALSE) -> ("FPGA VI Reference Out"=w347:T19, "error out"=w346:errorcluster)
      n164 = local write "Saving..."(FALSE ("Saving Data")) -> ()
      n165 = local write "Stop All"(FALSE ("Stop All")) -> ()
      n166 = local write "Retract Pump 1"(w340) -> ()
      n167 = local write "Retract Pump 3"(w340) -> ()
      n168 = local write "Index"(1.0 ("Index")) -> ()
      n169 = property on="Trap 1 ON" class="Bool (strict)"("Value"=w341) -> ()  [unwired: 2 in, 2 out]
      "Manipulating Trap" <- FALSE ("Manipulating Trap")
    }
    frame #1 {
      n170 = local read "Trap 2 (ON/OFF)"() -> (w351:bool)
      n171 = Wait (ms)(milliseconds to wait=u32 10) -> ()  [unwired: 1 out]
      n172 = property on="Trap 2 ON" class="Bool (strict)"("Val(Sgnl)"=w351) -> ()  [unwired: 2 in, 2 out]
    }
    frame #2 {
      n173 = local read "Scan Range (nm)"() -> (w355:dbl)
      n174 = xnode "Read/Write Control"("FPGA VI Reference In"=w362, "error in"=w361, "FPGA Controls  RF Box"=TRUE ("Direct RF Box  Communication")) -> ("FPGA VI Reference Out"=w360:T19, "error out"=w359:errorcluster)
      n175 = call "Update messages.vi"("Message to add"="UHR-Fleezers ready.", "Old message string"="") -> ("New message string"=w358:string)
      n176 = local write "Messages"(w358) -> ()
      n177 = property on="Scan Range (nm)" class="DigNum (strict)"("Val(Sgnl)"=w355) -> ()  [unwired: 2 in, 2 out]
    }
  }
  n178 = Subtract(x="BD 1 Frequency 1 (MHz)", y="BD 1 Frequency 2 (MHz)") -> (x-y=w209:dbl)
  n179 = Subtract(x="BD 2 Frequency 1 (MHz)", y="BD 2 Frequency 2 (MHz)") -> (x-y=w208:dbl)
  n180 = Square(x=w208) -> (x^2=w206:dbl)
  n181 = Square(x=w209) -> (x^2=w207:dbl)
  n182 = Add(x=w207, y=w206) -> (x+y=w205:dbl)
  n183 = Square Root(x=w205) -> (sqrt(x)=w204:dbl)
  n184 = local write "Trap Delta (MHz)"(w204) -> ()
  n185 = call "IMAQ Create"("Image Name"="APD 1 Image", "Image Type"=w119) -> ("New Image"=w118:T2)  [unwired: 3 in, 1 out]
  n186 = call "IMAQ Create"("Image Name"="APD 2 Image", "Image Type"=w119) -> ("New Image"=w117:T2)  [unwired: 3 in, 1 out]
  n187 = call "IMAQ Create"("Image Name"="Det. X Image", "Image Type"=w119) -> ("New Image"=w116:T2)  [unwired: 3 in, 1 out]
  n188 = call "IMAQ Create"("Image Name"="Det. Y Image", "Image Type"=w119) -> ("New Image"=w115:T2)  [unwired: 3 in, 1 out]
  n189 = Bundle("New Image"=w118, "New Image"=w117, "New Image"=w116, "New Image"=w115) -> (w114:T20)  [unwired: 1 in]
  n190 = call-poly "VISA Configure Serial Port"("VISA resource name"="Bottom  1 Harvard Syringe Pump Serial Port", "baud rate (9600)"=u32 115200, "stop bits (10: 1 bit)"=w58) -> ("VISA resource name out"=w54:refnum<visa-resource-name>, "error out"=w53:errorcluster)  [unwired: 4 in, 7 out]
  n191 = call-poly "VISA Configure Serial Port"("VISA resource name"="Top 3 Harvard Syringe Pump Serial Port", "baud rate (9600)"=u32 115200, "stop bits (10: 1 bit)"=w61) -> ("VISA resource name out"=w56:refnum<visa-resource-name>, "error out"=w55:errorcluster)  [unwired: 4 in, 7 out]
  n192 = call-poly "VISA Configure Serial Port"("VISA resource name"="Sample Chamber Stage Serial Port") -> ("VISA resource name out"=w128:refnum<visa-resource-name>, "error out"=w129:errorcluster)  [unwired: 5 in, 8 out]
  "Stage Control Serial Error" <- w129
  n193 = call-poly "VISA Configure Serial Port"("VISA resource name"="Center Harvard Syringe Pump Serial Port", "baud rate (9600)"=u32 115200, "stop bits (10: 1 bit)"=w112) -> ("VISA resource name out"=w109:refnum<visa-resource-name>, "error out"=w110:errorcluster)  [unwired: 4 in, 7 out]
  n194 = node-c288() -> (w139:T21)  [unwired: 4 out]
  n195 = node-c288() -> (w124:T21)  [unwired: 4 in]
  n196 = node-c288(i64 1 ("Period"), 1 ("Processor")) -> (w213:T21)  [unwired: 2 out]
  n197 = node-c288(2 ("Processor")) -> (w137:T21)  [unwired: 3 out]
  n198 = timed-loop "Mouse control: trap position (AOM deflection), set confocal spot from image" {
    tunnel: [w365] -> w220
    tunnel: w52 -> [w364]
    timing: w139 -> [_]
    timing-out: [_] -> w138
    stop <- w365 stop-if-true
    n199 = node-c288() -> ()  [unwired: 2 out]
    n200 = event shown="[0] \"Pane\": Mouse Down" {
      selector: _ -> [_ _]
      dyn-events: _ -> [_ _]
      timeout: _ -> [_ _]
      tunnel: w364 -> [w368 _]
      event Mouse Down {
        n201 = event-data() -> ("Time"=w370:u32, "Coords"=w369:T7, "Button"=w371:u16)  [unwired: 6 out]
        n202 = case shown="1" w371 {
          tunnel: w370 -> [_ _ w477]
          tunnel: w369 -> [_ w408 w475]
          tunnel: w368 -> [_ _ w473]
          frame 0, Default {
          }
          frame 1 {
            n203 = property on="APD 2" class="ImageControl"() -> ("Displayed Image Position"=w378:cluster{"Left":i32, "Top":i32})  [unwired: 2 in, 2 out]
            n204 = property on="APD 1" class="ImageControl"() -> ("Displayed Image Position"=w407:cluster{"Left":i32, "Top":i32})  [unwired: 2 in, 2 out]
            n205 = property on="Detection Laser X" class="ImageControl"() -> ("Displayed Image Position"=w404:cluster{"Left":i32, "Top":i32})  [unwired: 2 in, 2 out]
            n206 = property on="Detection Laser Y" class="ImageControl"() -> ("Displayed Image Position"=w403:cluster{"Left":i32, "Top":i32})  [unwired: 2 in, 2 out]
            n207 = property on="APD 2" class="ImageControl"() -> ("Displayed Image Size"=w377:cluster{"Width":u32, "Height":u32})  [unwired: 2 in, 2 out]
            n208 = property on="APD 1" class="ImageControl"() -> ("Displayed Image Size"=w405:cluster{"Width":u32, "Height":u32})  [unwired: 2 in, 2 out]
            n209 = property on="Detection Laser X" class="ImageControl"() -> ("Displayed Image Size"=w406:cluster{"Width":u32, "Height":u32})  [unwired: 2 in, 2 out]
            n210 = property on="Detection Laser Y" class="ImageControl"() -> ("Displayed Image Size"=w402:cluster{"Width":u32, "Height":u32})  [unwired: 2 in, 2 out]
            n211 = Unbundle By Name(w377) -> ("Width"=w374:u32, "Height"=w373:u32)
            n212 = Unbundle By Name(w378) -> ("Left"=w376:i32, "Top"=w375:i32)
            n213 = Unbundle By Name(w405) -> ("Width"=w399:u32, "Height"=w398:u32)
            n214 = Unbundle By Name(w406) -> ("Width"=w395:u32, "Height"=w394:u32)
            n215 = Unbundle By Name(w402) -> ("Width"=w391:u32, "Height"=w390:u32)
            n216 = Unbundle By Name(w407) -> ("Left"=w401:i32, "Top"=w400:i32)
            n217 = Unbundle By Name(w404) -> ("Left"=w397:i32, "Top"=w396:i32)
            n218 = Unbundle By Name(w403) -> ("Left"=w393:i32, "Top"=w392:i32)
            n219 = Bundle("Left"=w376, "Top"=w375, "Width"=w374, "Height"=w373) -> (w372:T24)  [unwired: 1 in]
            n220 = Bundle("Left"=w401, "Top"=w400, "Width"=w399, "Height"=w398) -> (w389:T24)  [unwired: 1 in]
            n221 = Bundle("Left"=w397, "Top"=w396, "Width"=w395, "Height"=w394) -> (w388:T24)  [unwired: 1 in]
            n222 = Bundle("Left"=w393, "Top"=w392, "Width"=w391, "Height"=w390) -> (w387:T24)  [unwired: 1 in]
            n223 = Build Cluster Array(w372, w389, w388, w387) -> (w386:T25)
            n224 = for {
              tunnel: w408 -> [w419]
              tunnel: w386 -> [w420] mode=indexing
              shift-right: [w417] -> w384
              shift-left: TRUE -> [w418]
              shift-right: [w416] -> w382
              shift-left: _ -> [w412]
              shift-right: [w415] -> w381
              shift-left: _ -> [w411]
              shift-right: [w414] -> w380
              shift-left: _ -> [w410]
              shift-right: [w413] -> w379
              shift-left: _ -> [w409]
              n225 = case shown="True" w418 {
                selector: w418 -> [w425 _]
                tunnel: w420 -> [_ w434]
                tunnel: w419 -> [_ w432]
                tunnel: [w425 w430] -> w417
                tunnel: [w424 w429] -> w416
                tunnel: [w423 w428] -> w415
                tunnel: [w422 w427] -> w414
                tunnel: [w421 w426] -> w413
                tunnel: w412 -> [w424 _]
                tunnel: w411 -> [w423 _]
                tunnel: w410 -> [w422 _]
                tunnel: w409 -> [w421 _]
                frame False {
                }
                frame True {
                  n226 = Unbundle(w434) -> (w433:T24)
                  n227 = call "isclickinwindow.vi"("Image Param"=w433, "Point32"=w432) -> ("4 Y"=w426:i32, "3 Height"=w427:i32, "2 X"=w428:i32, "1 Width"=w429:i32, "In image?"=w431:bool)  [unwired: 1 in]
                  n228 = Not(x=w431) -> (.not. x?=w430:bool)
                }
              }
            }
            n229 = Not(x=w384) -> (.not. x?=w383:bool)
            n230 = case shown="True" w383 {
              tunnel: w381 -> [_ w448]
              tunnel: w379 -> [_ w447]
              tunnel: w382 -> [_ w446]
              tunnel: w380 -> [_ w445]
              frame False {
              }
              frame True {
                w435 = FALSE ("Get Point")
                n231 = local read "Scan lines (y)"() -> (w450:u64)
                n232 = disable-structure shown="Disabled" {
                  frame Disabled {
                  }
                  frame Enabled {
                  }
                }
                n233 = local read "Actual MCL Inc (V)"() -> (w444:dbl)
                n234 = local read "Scan steps (MCL)"() -> (w449:u64)
                n235 = Divide "Y Pix/step"(x=w445, y=w450) -> (x/y=w457:dbl)
                n236 = Divide "Y V/pix"(x=w444, y=w457) -> (x/y=w456:dbl)
                n237 = Divide "Y half step offset"(x=w444, y=2.0) -> (x/y=w458:dbl)
                n238 = Divide "X pix/step"(x=w446, y=w449) -> (x/y=w455:dbl)
                n239 = Negate(x=w458) -> (-x=w459:dbl)
                n240 = local read "Initial Y"() -> (w465:dbl)
                n241 = Multiply(x=w447, y=w456) -> (x*y=w466:dbl)
                n242 = Divide "X half step offset"(x=w444, y=2.0) -> (x/y=w452:dbl)
                n243 = Divide "X V/pix"(x=w444, y=w455) -> (x/y=w454:dbl)
                n244 = Multiply(x=w444, y=w449) -> (x*y=w461:dbl)
                n245 = Compound Arithmetic op=ADD(w459, w466, w465) -> (w436:dbl)
                "Pointer Y (V)" <- w436
                n246 = Multiply(x=w454, y=w448) -> (x*y=w463:dbl)
                n247 = Negate(x=w452) -> (-x=w451:dbl)
                n248 = local read "Initial X"() -> (w464:dbl)
                n249 = Negate(x=w463) -> (-x=w462:dbl)
                n250 = Compound Arithmetic op=ADD(w451, w461, w464, w462) -> (w437:dbl)
                "Pointer X (V)" <- w437
                n251 = case shown="True" "Set High F Confocal Spot (X-Y)" {
                  tunnel: w437 -> [_ w467]
                  tunnel: w436 -> [_ w468]
                  frame False {
                  }
                  frame True {
                    "Confocal Y 2 (V)" <- w468
                    "Confocal X 2 (V)" <- w467
                  }
                }
                n252 = Or(x="Set X Only", y="Set Confocal Spot (X-Y)") -> (x .or. y?=w440:bool)
                n253 = Or(x="Set Confocal Spot (X-Y)", y="Set Y Only") -> (x .or. y?=w439:bool)
                n254 = case shown="True" w440 {
                  tunnel: w437 -> [_ w469]
                  frame False {
                  }
                  frame True {
                    n255 = property on="AO2" class="Slide (strict)"("Val(Sgnl)"=w469) -> ()  [unwired: 2 in, 2 out]
                    "Confocal X 1 (V)" <- w469
                  }
                }
                n256 = case shown="True" w439 {
                  tunnel: w436 -> [_ w470]
                  frame False {
                  }
                  frame True {
                    n257 = property on="AO1" class="Slide (strict)"("Val(Sgnl)"=w470) -> ()  [unwired: 2 in, 2 out]
                    "Confocal Y 1 (V)" <- w470
                  }
                }
                n258 = local write "Set High F Confocal Spot (X-Y)"(w435) -> ()
                n259 = local write "Set Confocal Spot (X-Y)"(w435) -> ()
                n260 = local write "Set X Only"(w435) -> ()
                n261 = local write "Set Y Only"(w435) -> ()
              }
            }
          }
          frame 3 {
            n262 = local read "BD 2 Frequency 1 (MHz)"() -> (w471:dbl)
            n263 = local read "BD 1 Frequency 1 (MHz)"() -> (w472:dbl)
            n264 = local write "Manipulating Trap"(TRUE ("Manipulating Trap")) -> ()
            n265 = local write "Coords"(T7 {"Horizontal"=0, "Vertical"=0} ("Coords")) -> ()
